vi "NM GlobalTest.vi"() -> ()   [LabVIEW 2010] (continued)
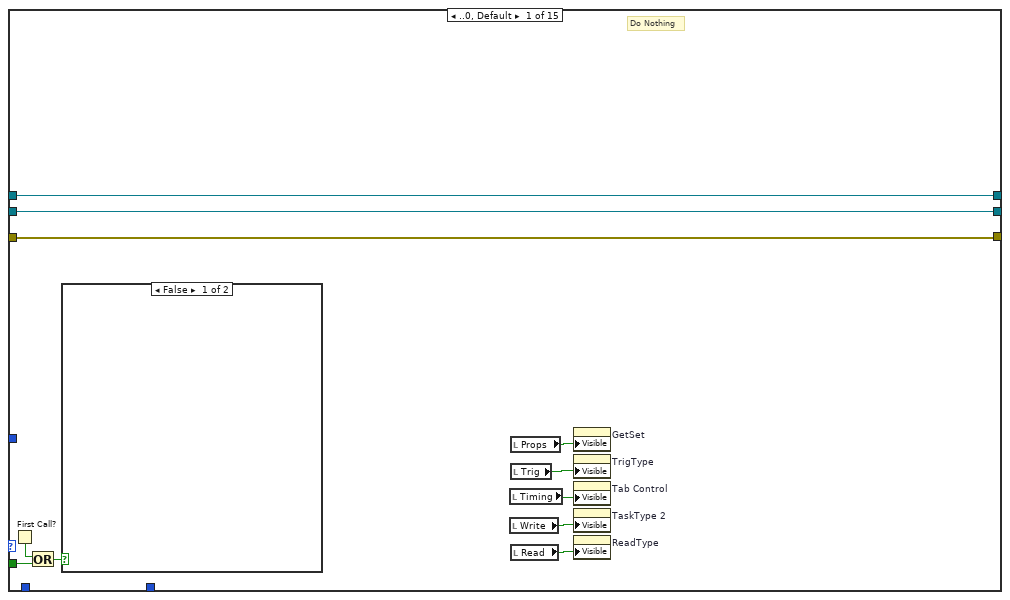
[diagram p2: hidden frame]
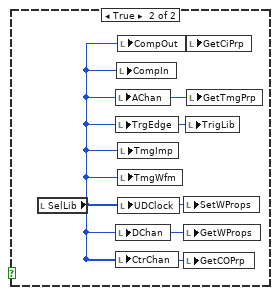
[diagram p3: hidden frame]
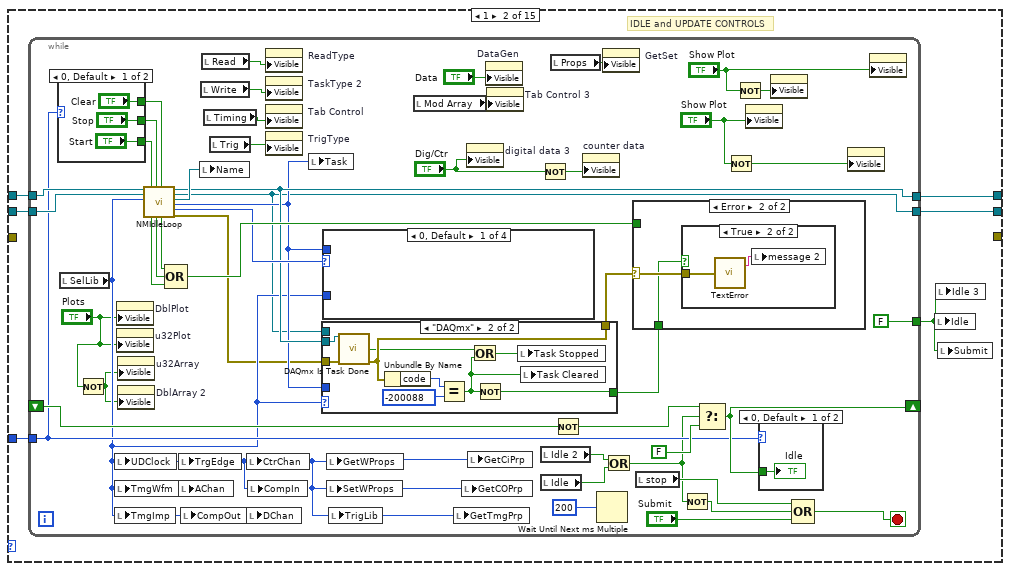
[diagram p4: hidden frame]
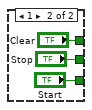
[diagram p5: hidden frame]
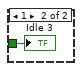
[diagram p6: hidden frame]
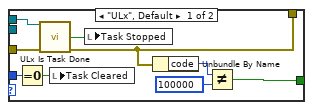
[diagram p7: hidden frame]
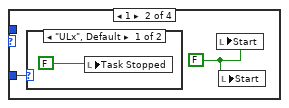
[diagram p8: hidden frame]
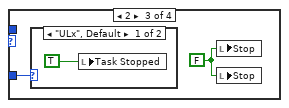
[diagram p10: hidden frame]
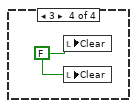
[diagram p12: hidden frame]
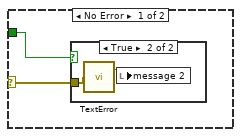
[diagram p13: hidden frame]
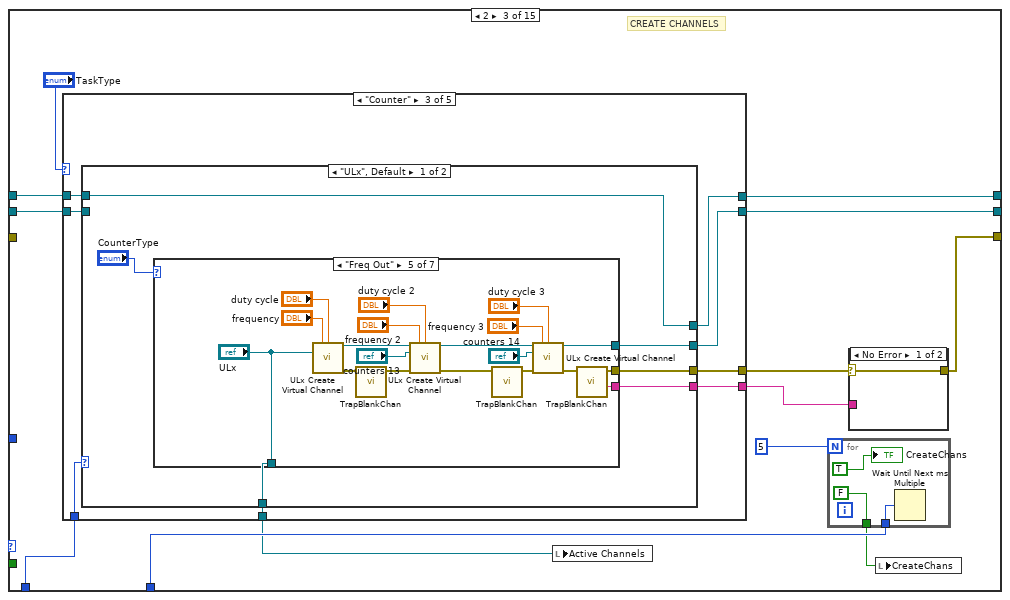
[diagram p16: hidden frame]
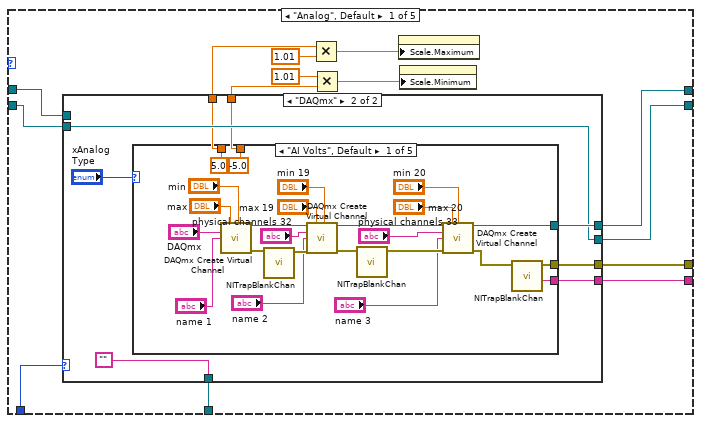
[diagram p17: hidden frame]
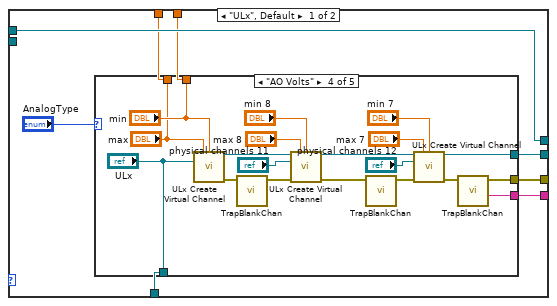
[diagram p18: hidden frame]
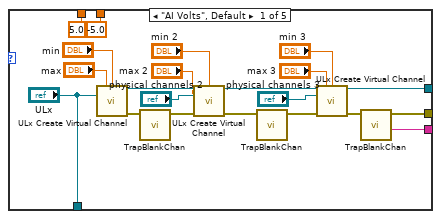
[diagram p19: hidden frame]
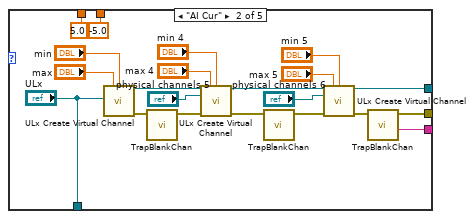
[diagram p20: hidden frame]
                                }
                                }
                                "Rate" <- w4838
                              }
                              frame 6 {
                                n979 = case shown="\"DAQmx\"" w4864 {
                                tunnel: w4863 -> [w4865 w4872]
                                tunnel: [w4865 w4871] -> w4862
                                tunnel: w4861 -> [w4866 w4870]
                                tunnel: [w4866 w4870] -> w4860
                                tunnel: w4859 -> [w4867 w4869]
                                tunnel: [w4867 w4868] -> w4858
                                frame "ULx", Default {
                                }
                                frame "DAQmx" {
                                n980 = property class="DAQmx Timing"(reference=w4869, error in=w4872) -> (reference out=w4868:refnum<k21>, error out=w4871:errorcluster, "SampClk.UnderflowBehavior"=→"SampClk.UnderflowBehavior":i32)
                                }
                                }
                              }
                            }
                          }
                        }
                        frame "AI" {
                          n981 = case shown="True" "Units" {
                            tunnel: w4905 -> [w4908 w4915]
                            tunnel: w4904 -> [w4907 w4914]
                            tunnel: w4903 -> [w4906 w4913]
                            tunnel: w4902 -> [_ w4912]
                            tunnel: [w4908 w4911] -> w4901
                            tunnel: [w4907 w4910] -> w4900
                            tunnel: [w4906 w4909] -> w4899
                            frame False {
                            }
                            frame True {
                              n982 = stacked-sequence {
                                seq-local: [w4919 _] -> [_ w4931]
                                seq-local: [w4918 _] -> [_ w4930]
                                seq-local: [w4917 _] -> [_ w4929]
                                tunnel: w4915 -> [w4922 _]
                                tunnel: w4914 -> [w4921 _]
                                tunnel: w4913 -> [w4920 _]
                                tunnel: w4912 -> [w4916 w4935]
                                tunnel: [_ w4934] -> w4911
                                tunnel: [_ w4933] -> w4910
                                tunnel: [_ w4932] -> w4909
                                frame #0 {
                                n983 = case shown="\"ULx\", Default" w4916 {
                                tunnel: w4921 -> [w4923 w4928]
                                tunnel: [w4924 w4927] -> w4917
                                tunnel: [w4923 w4928] -> w4918
                                tunnel: [w4925 w4926] -> w4919
                                tunnel: w4922 -> [w4925 w4926]
                                tunnel: w4920 -> [w4924 w4927]
                                frame "ULx", Default {
                                }
                                frame "DAQmx" {
                                }
                                }
                                }
                                frame #1 {
                                n984 = case shown="\"ULx\", Default" w4935 {
                                tunnel: w4930 -> [w4940 w4947]
                                tunnel: [w4936 w4945] -> w4932
                                tunnel: [w4937 w4947] -> w4933
                                tunnel: [w4941 w4943] -> w4934
                                tunnel: w4931 -> [w4941 w4944]
                                tunnel: w4929 -> [w4938 w4946]
                                frame "ULx", Default {
                                n985 = call "TempUnits.vi"("error in (no error)"=w4938, "task in"=w4940) -> ("error out"=w4936:errorcluster, "Temp.Units"=→"Channel.AI.Temp.Units":i32, "task out"=w4937:refnum<k24>)  [unwired: 1 in]
                                }
                                frame "DAQmx" {
                                n986 = property class="DAQmx Channel"(reference=w4944, error in=w4946) -> (reference out=w4943:refnum<k21>, error out=w4945:errorcluster, "AI.Temp.Units"=→"DAQmx AI.Temp.Units":i32)
                                }
                                }
                                }
                              }
                            }
                          }
                        }
                        frame "CI" {
                          n987 = stacked-sequence {
                            seq-local: [w4957 _] -> [_ w4974]
                            seq-local: [w4955 _] -> [_ w4973]
                            seq-local: [w4956 _] -> [_ w4972]
                            tunnel: w4954 -> [w4960 _]
                            tunnel: w4953 -> [w4955 _]
                            tunnel: w4952 -> [w4959 _]
                            tunnel: [_ w4977] -> w4951
                            tunnel: [_ w4976] -> w4950
                            tunnel: [_ w4975] -> w4949
                            tunnel: w4948 -> [w4958 w4971]
                            frame #0 {
                              n988 = case shown="\"ULx\", Default" w4958 {
                                tunnel: w4960 -> [w4961 w4969]
                                tunnel: w4959 -> [w4962 w4968]
                                tunnel: [w4962 w4967] -> w4957
                                tunnel: [w4961 w4966] -> w4956
                                frame "ULx", Default {
                                }
                                frame "DAQmx" {
                                n989 = property class="DAQmx Channel"(reference=w4968, error in=w4969) -> (reference out=w4967:refnum<k21>, error out=w4966:errorcluster, "CI.Max"=→"Max":dbl, "CI.Min"=→"Min":dbl, "CI.MeasType"=→"MeasType":i32)
                                }
                              }
                            }
                            frame #1 {
                              n990 = case shown="\"ULx\", Default" w4971 {
                                tunnel: ["CIType" "GetmxCIPrp"] -> w4970
                                frame "ULx", Default {
                                }
                                frame "DAQmx" {
                                }
                              }
                              n991 = case shown="\"Edges\"" w4970 {
                                tunnel: w4972 -> [w4986 w5010 w5038 w5077]
                                tunnel: w4973 -> [w4984 w5011 w5035 w5076]
                                tunnel: [w4981 w5009 w5036 w5075] -> w4977
                                tunnel: [w4985 w5007 w5037 w5073] -> w4976
                                tunnel: [w4983 w5008 w5034 w5074] -> w4975
                                tunnel: w4971 -> [w4982 w5012 w5033 w5072]
                                tunnel: w4974 -> [w4980 w5006 w5032 w5071]
                                frame "Frequency", Default {
                                n992 = case shown="\"ULx\", Default" w4982 {
                                tunnel: w4986 -> [w4992 w5005]
                                tunnel: [w4990 w4996] -> w4985
                                tunnel: w4984 -> [w4993 w5003]
                                tunnel: [w4991 w5003] -> w4983
                                tunnel: w4980 -> [w4994 w5004]
                                tunnel: [w4994 w4995] -> w4981
                                frame "ULx", Default {
                                n993 = call "CIFreqProps.vi"("task in"=w4993, "error in (no error)"=w4992) -> ("task out"=w4991:refnum<k24>, "StartingEdge"=→"StartingEdge":i32, "Units"=→"Units":i32, "error out"=w4990:errorcluster, "MeasurementTime"=→"MeasurementTime":dbl)  [unwired: 1 in]
                                }
                                frame "DAQmx" {
                                n994 = property class="DAQmx Channel"(reference=w5004, error in=w5005) -> (reference out=w4995:refnum<k21>, error out=w4996:errorcluster, "CI.Freq.Units"=→"Units":i32, "CI.Freq.Term"=→"Term":tag, "CI.Freq.StartingEdge"=→"StartingEdge":i32, "CI.Freq.MeasMeth"=→"Method":i32, "CI.Freq.MeasTime"=→"MeasTime":dbl, "CI.Freq.Div"=→"Divisor":u32)
                                }
                                }
                                }
                                frame "Period" {
                                n995 = case shown="\"ULx\", Default" w5012 {
                                tunnel: w5010 -> [w5017 w5031]
                                tunnel: [w5016 w5030] -> w5007
                                tunnel: w5011 -> [w5019 w5027]
                                tunnel: [w5018 w5027] -> w5008
                                tunnel: w5006 -> [w5020 w5029]
                                tunnel: [w5020 w5028] -> w5009
                                frame "ULx", Default {
                                n996 = call "CIPeriodProps.vi"("task in"=w5019, "error in (no error)"=w5017) -> ("task out"=w5018:refnum<k24>, "StartingEdge"=→"StartingEdge":i32, "Units"=→"Units":i32, "error out"=w5016:errorcluster, "MeasurementTime"=→"MeasurementTime":dbl)  [unwired: 1 in]
                                }
                                frame "DAQmx" {
                                n997 = property class="DAQmx Channel"(reference=w5029, error in=w5031) -> (reference out=w5028:refnum<k21>, error out=w5030:errorcluster, "CI.Period.Units"=→"Units":i32, "CI.Period.Term"=→"Term":tag, "CI.Period.StartingEdge"=→"StartingEdge":i32, "CI.Period.MeasMeth"=→"Method":i32, "CI.Period.MeasTime"=→"MeasTime":dbl, "CI.Period.Div"=→"Divisor":u32)
                                }
                                }
                                }
                                frame "Edges" {
                                n998 = case shown="\"ULx\", Default" w5033 {
                                tunnel: w5038 -> [w5059 w5070]
                                tunnel: [w5041 w5068] -> w5037
                                tunnel: w5035 -> [w5060 w5066]
                                tunnel: [w5042 w5066] -> w5034
                                tunnel: w5032 -> [w5061 w5069]
                                tunnel: [w5061 w5067] -> w5036
                                frame "ULx", Default {
                                n999 = call "CIEdgesProps.vi"("task in"=w5060, "error in (no error)"=w5059) -> ("task out"=w5048:refnum<k24>, "Edge"=→"Edge":i32, "InitialCount"=→"InitialCount":u32, "error out"=w5047:errorcluster, "Direction"=→"MccDirection":i32, "Gate Function"=→"Gate Function":i32)
                                n1000 = call "CtrCntrl.vi"("error in (no error)"=w5047, ".NET Refnum"=w5048) -> ("InvertGate"=→"InvertGate":bool, "Recycle"=→"Recycle":bool, "error out"=w5043:errorcluster, ".NET Refnum 2"=w5044:refnum<k24>, "OutputVal1"=→"Val 1":u64, "MinLimit"=→"Min":u64, "OutputVal0"=→"Val 0":u64, "MaxLimit"=→"Max":u64, "OutputOn"=→"Output":bool, "RangeLimitOn"=→"Range Limit":bool)
                                n1001 = call "CtrProps.vi"("error in (no error)"=w5043, ".NET Refnum 2"=w5044) -> ("InitialState"=→"InitialState":i32, "ClearOnRead"=→"ClearOnRead":bool, "error out"=w5041:errorcluster, ".NET Refnum"=w5042:refnum<k24>)  [unwired: 6 in]
                                }
                                frame "DAQmx" {
                                n1002 = property class="DAQmx Channel"(reference=w5069, error in=w5070) -> (reference out=w5067:refnum<k21>, error out=w5068:errorcluster, "CI.CountEdges.Term"=→"Term":tag, "CI.CountEdges.Dir"=→"Direction":i32, "CI.CountEdges.InitialCnt"=→"InitialCnt":u32, "CI.CountEdges.ActiveEdge"=→"ActiveEdge":i32)
                                }
                                }
                                }
                                frame "Encoder" {
                                n1003 = case shown="\"ULx\", Default" w5072 {
                                tunnel: w5077 -> [w5086 w5100]
                                tunnel: [w5078 w5099] -> w5073
                                tunnel: w5076 -> [w5085 w5098]
                                tunnel: [w5079 w5098] -> w5074
                                tunnel: w5071 -> [w5087 w5102]
                                tunnel: [w5087 w5101] -> w5075
                                frame "ULx", Default {
                                n1004 = call "CIEncoderProps.vi"("task in"=w5085, "error in (no error)"=w5086) -> ("Units"=→"Units":i32, "DecodingType"=→"DecodingType":i32, "task out"=w5079:refnum<k24>, "PulsesPerRevolution"=→"PulsesPerRev":i32, "InitialAngle"=→"InitialAngle":dbl, "ZIndexMode"=→"ZIndexMode":i32, "error out"=w5078:errorcluster)  [unwired: 2 in]
                                }
                                frame "DAQmx" {
                                n1005 = property class="DAQmx Channel"(reference=w5102, error in=w5100) -> (reference out=w5101:refnum<k21>, error out=w5099:errorcluster, "CI.AngEncoder.Units"=→"Units":i32, "CI.AngEncoder.PulsesPerRev"=→"PulsesPerRev":u32, "CI.AngEncoder.InitialAngle"=→"InitialAngle":dbl, "CI.Encoder.DecodingType"=→"Type":i32, "CI.Encoder.AInputTerm"=→"AInputTerm":tag, "CI.Encoder.BInputTerm"=→"BInputTerm":tag, "CI.Encoder.ZInputTerm"=→"ZInputTerm":tag, "CI.Encoder.ZIndexEnable"=→"ZIndex":bool, "CI.Encoder.ZIndexVal"=→"Value":dbl, "CI.Encoder.ZIndexPhase"=→"Phase":i32)
                                }
                                }
                                }
                              }
                            }
                          }
                        }
                        frame "CO" {
                          n1006 = case shown="\"ULx\", Default" w5103 {
                            tunnel: w5108 -> [w5119 w5130]
                            tunnel: [w5116 w5121] -> w5104
                            tunnel: [w5117 w5130] -> w5105
                            tunnel: [w5120 w5122] -> w5106
                            tunnel: w5109 -> [w5120 w5127]
                            tunnel: w5107 -> [w5118 w5126]
                            frame "ULx", Default {
                              n1007 = call "COPulseProps.vi"("task in"=w5119, "error in (no error)"=w5118) -> ("DutyCycle"=→"DutyCycle":dbl, "HighTicks"=→"HighTicks":u32, "HighTime"=→"HighTime":dbl, "task out"=w5117:refnum<k24>, "LowTicks"=→"LowTicks":u32, "Frequency"=→"Frequency":dbl, "LowTime"=→"LowTime":dbl, "error out"=w5116:errorcluster)  [unwired: 1 in]
                            }
                            frame "DAQmx" {
                              n1008 = property class="DAQmx Channel"(reference=w5127, error in=w5126) -> (reference out=w5124:refnum<k21>, error out=w5123:errorcluster, "CO.OutputType"=→"OutputType":i32, "CO.Pulse.IdleState"=→"IdleState":i32)
                              n1009 = case shown="\"Freq\", Default" "mxCOType" {
                                tunnel: w5124 -> [w5138 w5143 w5152]
                                tunnel: w5123 -> [w5137 w5146 w5153]
                                tunnel: [w5136 w5144 w5151] -> w5122
                                tunnel: [w5135 w5145 w5150] -> w5121
                                frame "Freq", Default {
                                n1010 = property class="DAQmx Channel"(reference=w5138, error in=w5137) -> (reference out=w5136:refnum<k21>, error out=w5135:errorcluster, "CO.Pulse.DutyCyc"=→"DutyCyc":dbl, "CO.Pulse.Freq.Units"=→"Freq.Units":i32, "CO.Pulse.Freq"=→"Freq":dbl, "CO.Pulse.Freq.InitialDelay"=→"Freq.Delay":dbl)
                                }
                                frame "Time" {
                                n1011 = property class="DAQmx Channel"(reference=w5143, error in=w5146) -> (reference out=w5144:refnum<k21>, error out=w5145:errorcluster, "CO.Pulse.Time.Units"=→"Time.Units":i32, "CO.Pulse.HighTime"=→"HighTime":dbl, "CO.Pulse.LowTime"=→"LowTime":dbl, "CO.Pulse.Time.InitialDelay"=→"Time.Delay":dbl)
                                }
                                frame "Ticks" {
                                n1012 = property class="DAQmx Channel"(reference=w5152, error in=w5153) -> (reference out=w5151:refnum<k21>, error out=w5150:errorcluster, "CO.Pulse.HighTicks"=→"HighTicks":u32, "CO.Pulse.LowTicks"=→"LowTicks":u32, "CO.Pulse.Ticks.InitialDelay"=→"Ticks.Delay":u32)
                                }
                              }
                            }
                          }
                        }
                      }
                    }
                  }
                }
                frame "Set Properties" {
                  n1013 = case shown="\"Write\"" "SetLev" {
                    tunnel: w5161 -> [w5169 w5257 _ w5379 _ w5475 w5725]
                    tunnel: w5160 -> [w5167 w5263 w5371 w5376 w5472 w5480 w5722]
                    tunnel: [w5166 w5260 w5371 w5375 w5472 w5479 w5720] -> w5159
                    tunnel: [w5165 w5259 w5370 w5374 w5471 w5477 w5719] -> w5158
                    tunnel: w5157 -> [w5164 w5262 w5370 w5377 w5471 w5474 w5723]
                    tunnel: w5156 -> [w5163 w5261 w5369 w5378 w5470 w5473 w5724]
                    tunnel: [w5162 w5258 w5369 w5373 w5470 w5478 w5718] -> w5154
                    frame "Read", Default {
                      n1014 = for {
                        N: 3 -> [_]
                        tunnel: w5169 -> [w5175]
                        shift-right: [w5178] -> w5166
                        shift-left: w5167 -> [w5172]
                        shift-right: [w5177] -> w5165
                        shift-left: w5164 -> [w5171]
                        shift-right: [w5176] -> w5162
                        shift-left: w5163 -> [w5170]
                        i -> [w5174]
                        n1015 = case shown="0, Default" w5174 {
                          tunnel: [w5179 w5183 w5187] -> w5173
                          frame 0, Default {
                            n1016 = Select(t=1, s="Auto", f=0) -> (s? t:f=w5179:i32)
                          }
                          frame 1 {
                            n1017 = Select(t=2, s="OWrite", f=0) -> (s? t:f=w5183:i32)
                          }
                          frame 2 {
                            n1018 = Select(t=3, s="ReadAll 2", f=0) -> (s? t:f=w5187:i32)
                          }
                        }
                        n1019 = case shown="3" w5173 {
                          tunnel: w5172 -> [w5193 w5202 w5217 w5244]
                          tunnel: w5171 -> [w5192 w5201 w5221 w5243]
                          tunnel: w5170 -> [w5191 w5200 w5223 w5242]
                          tunnel: [w5193 w5199 w5216 w5240] -> w5178
                          tunnel: [w5192 w5198 w5220 w5241] -> w5177
                          tunnel: [w5191 w5197 w5222 w5239] -> w5176
                          tunnel: w5175 -> [_ w5196 w5218 w5237]
                          frame 0, Default {
                          }
                          frame 1 {
                            n1020 = case shown="\"ULx\", Default" w5196 {
                              tunnel: w5201 -> [w5203 w5214]
                              tunnel: [w5205 w5212] -> w5197
                              tunnel: [w5204 w5214] -> w5198
                              tunnel: [w5208 w5211] -> w5199
                              tunnel: w5202 -> [w5208 w5210]
                              tunnel: w5200 -> [w5206 w5213]
                              tunnel: "Read.AutoStart" -> [w5207 w5209]
                              frame "ULx", Default {
                                n1021 = call "SetReadAutostart.vi"("error in (no error)"=w5206, "Read.AutoStart"=w5207, "task in"=w5203) -> ("error out"=w5205:errorcluster, "task out"=w5204:refnum<k24>)
                              }
                              frame "DAQmx" {
                                n1022 = property class="DAQmx Read"(reference=w5210, error in=w5213, "AutoStart"=w5209) -> (reference out=w5211:refnum<k21>, error out=w5212:errorcluster)
                              }
                            }
                            n1023 = local write "Auto"(FALSE ("Auto")) -> ()
                          }
                          frame 2 {
                            n1024 = case shown="\"ULx\", Default" w5218 {
                              tunnel: w5223 -> [w5224 w5233]
                              tunnel: [w5224 w5232] -> w5222
                              tunnel: w5221 -> [w5225 w5229]
                              tunnel: [w5225 w5229] -> w5220
                              tunnel: w5217 -> [w5226 w5231]
                              tunnel: [w5226 w5230] -> w5216
                              tunnel: "Overwrite" -> [_ w5228]
                              frame "ULx", Default {
                              }
                              frame "DAQmx" {
                                n1025 = case shown="False" w5228 {
                                tunnel: [w5234 w5235] -> w5227
                                frame False {
                                w5234 = 10159 items=["Overwrite Unread Samples"=10252, "Do Not Overwrite Unread Samples"=10159] ("OverWrite")
                                }
                                frame True {
                                w5235 = 10252 items=["Overwrite Unread Samples"=10252, "Do Not Overwrite Unread Samples"=10159] ("OverWrite")
                                }
                                }
                                n1026 = property class="DAQmx Read"(reference=w5231, error in=w5233, "OverWrite"=w5227) -> (reference out=w5230:refnum<k21>, error out=w5232:errorcluster)
                              }
                            }
                            n1027 = local write "OWrite"(FALSE ("Auto 2")) -> ()
                          }
                          frame 3 {
                            n1028 = case shown="\"ULx\", Default" w5237 {
                              tunnel: w5242 -> [w5249 w5256]
                              tunnel: [w5248 w5255] -> w5239
                              tunnel: w5243 -> [w5247 w5252]
                              tunnel: [w5246 w5252] -> w5241
                              tunnel: w5244 -> [w5250 w5254]
                              tunnel: [w5250 w5253] -> w5240
                              tunnel: "ReadAllAvailSamp" -> [w5245 w5251]
                              frame "ULx", Default {
                                n1029 = call "SetReadAllData.vi"("error in (no error)"=w5249, "Read.AllData"=w5245, "task in"=w5247) -> ("error out"=w5248:errorcluster, "task out"=w5246:refnum<k24>)
                              }
                              frame "DAQmx" {
                                n1030 = property class="DAQmx Read"(reference=w5254, error in=w5256, "ReadAllAvailSamp"=w5251) -> (reference out=w5253:refnum<k21>, error out=w5255:errorcluster)
                              }
                            }
                            n1031 = local write "ReadAll 2"(FALSE ("ReadAll 2")) -> ()
                          }
                        }
                      }
                    }
                    frame "Write" {
                      n1032 = for {
                        N: 4 -> [_]
                        shift-right: [w5269] -> w5260
                        shift-left: w5263 -> [w5271]
                        shift-right: [w5268] -> w5259
                        shift-left: w5262 -> [w5270]
                        shift-right: [w5272] -> w5258
                        shift-left: w5261 -> [w5273]
                        tunnel: w5257 -> [w5265]
                        i -> [w5267]
                        n1033 = case shown="0, Default" w5267 {
                          tunnel: [w5274 w5278 w5282 w5286] -> w5266
                          frame 0, Default {
                            n1034 = Select(t=1, s="WrtPos", f=0) -> (s? t:f=w5274:i32)
                          }
                          frame 1 {
                            n1035 = Select(t=2, s="Reg", f=0) -> (s? t:f=w5278:i32)
                          }
                          frame 2 {
                            n1036 = Select(t=3, s="Rel", f=0) -> (s? t:f=w5282:i32)
                          }
                          frame 3 {
                            n1037 = Select(t=4, s="Offset 3", f=0) -> (s? t:f=w5286:i32)
                          }
                        }
                        n1038 = case shown="4" w5266 {
                          tunnel: w5273 -> [w5290 w5301 w5319 w5339 w5356]
                          tunnel: [w5290 w5300 w5314 w5335 w5352] -> w5272
                          tunnel: w5271 -> [w5292 w5299 w5318 w5341 w5358]
                          tunnel: w5270 -> [w5291 w5298 w5317 w5340 w5357]
                          tunnel: [w5292 w5297 w5316 w5337 w5354] -> w5269
                          tunnel: [w5291 w5296 w5315 w5336 w5353] -> w5268
                          tunnel: w5265 -> [_ w5295 w5313 w5338 w5355]
                          frame 0, Default {
                          }
                          frame 1 {
                            n1039 = case shown="\"DAQmx\"" w5295 {
                              tunnel: w5298 -> [w5304 w5310]
                              tunnel: [w5305 w5309] -> w5300
                              tunnel: [w5303 w5310] -> w5296
                              tunnel: [w5307 w5308] -> w5297
                              tunnel: w5299 -> [w5307 w5308]
                              tunnel: w5301 -> [w5306 w5309]
                              tunnel: "CurrentWrite\nPosition (ULx)" -> [w5302 _]
                              frame "ULx", Default {
                                n1040 = call "SetCurWrtPos.vi"("error in (no error)"=w5306, "CurrentWritePosition"=w5302, "task in"=w5304) -> ("error out"=w5305:errorcluster, "task out"=w5303:refnum<k24>)
                              }
                              frame "DAQmx" {
                              }
                            }
                            n1041 = local write "WrtPos"(FALSE ("WrtPos")) -> ()
                          }
                          frame 2 {
                            n1042 = case shown="\"ULx\", Default" w5313 {
                              tunnel: w5319 -> [w5322 w5331]
                              tunnel: [w5321 w5327] -> w5314
                              tunnel: w5317 -> [w5323 w5330]
                              tunnel: [w5320 w5330] -> w5315
                              tunnel: w5318 -> [w5325 w5329]
                              tunnel: [w5325 w5328] -> w5316
                              tunnel: "Regenerate" -> [w5324 w5326]
                              frame "ULx", Default {
                                n1043 = call "SetWrtRegen.vi"("error in (no error)"=w5322, "Regenerate"=w5324, "task in"=w5323) -> ("error out"=w5321:errorcluster, "task out"=w5320:refnum<k24>)
                              }
                              frame "DAQmx" {
                                n1044 = case shown="True" w5326 {
                                tunnel: [w5333 w5334] -> w5332
                                frame False {
                                w5333 = 10158 items=["Allow Regeneration"=10097, "Do Not Allow Regeneration"=10158] ("RegenMode")
                                }
                                frame True {
                                w5334 = 10097 items=["Allow Regeneration"=10097, "Do Not Allow Regeneration"=10158] ("RegenMode")
                                }
                                }
                                n1045 = property class="DAQmx Write"(reference=w5329, error in=w5331, "RegenMode"=w5332) -> (reference out=w5328:refnum<k21>, error out=w5327:errorcluster)
                              }
                            }
                            n1046 = local write "Reg"(FALSE ("Reg")) -> ()
                          }
                          frame 3 {
                            n1047 = case shown="\"DAQmx\"" w5338 {
                              tunnel: w5339 -> [w5343 w5351]
                              tunnel: [w5343 w5347] -> w5335
                              tunnel: w5340 -> [w5342 w5350]
                              tunnel: [w5342 w5350] -> w5336
                              tunnel: w5341 -> [w5344 w5349]
                              tunnel: [w5344 w5348] -> w5337
                              frame "ULx", Default {
                              }
                              frame "DAQmx" {
                                n1048 = property class="DAQmx Write"(reference=w5349, error in=w5351, "RelativeTo"="RelativeTo") -> (reference out=w5348:refnum<k21>, error out=w5347:errorcluster)
                                n1049 = local write "Rel"(FALSE ("Rel")) -> ()
                              }
                            }
                          }
                          frame 4 {
                            n1050 = case shown="\"DAQmx\"" w5355 {
                              tunnel: w5356 -> [w5360 w5368]
                              tunnel: [w5360 w5364] -> w5352
                              tunnel: w5357 -> [w5359 w5367]
                              tunnel: [w5359 w5367] -> w5353
                              tunnel: w5358 -> [w5361 w5366]
                              tunnel: [w5361 w5365] -> w5354
                              frame "ULx", Default {
                              }
                              frame "DAQmx" {
                                n1051 = property class="DAQmx Write"(reference=w5366, error in=w5368, "Offset"="Offset") -> (reference out=w5365:refnum<k21>, error out=w5364:errorcluster)
                                n1052 = local write "Offset 3"(FALSE ("Rel")) -> ()
                              }
                            }
                          }
                        }
                      }
                    }
                    frame "Trigger" {
                    }
                    frame "Timing" {
                      n1053 = for {
                        N: 4 -> [_]
                        tunnel: w5379 -> [w5388]
                        shift-right: [w5384] -> w5375
                        shift-left: w5376 -> [w5385]
                        shift-right: [w5383] -> w5374
                        shift-left: w5377 -> [w5386]
                        shift-right: [w5382] -> w5373
                        shift-left: w5378 -> [w5387]
                        i -> [w5381]
                        n1054 = case shown="0, Default" w5381 {
                          tunnel: [w5389 w5393 w5397 w5401] -> w5380
                          frame 0, Default {
                            n1055 = Select(t=1, s="BurstIO 3", f=0) -> (s? t:f=w5389:i32)
                          }
                          frame 1 {
                            n1056 = Select(t=2, s="SingleIO 3", f=0) -> (s? t:f=w5393:i32)
                          }
                          frame 2 {
                            n1057 = Select(t=3, s="DIWord", f=0) -> (s? t:f=w5397:i32)
                          }
                          frame 3 {
                            n1058 = Select(t=4, s="DOWord 2", f=0) -> (s? t:f=w5401:i32)
                          }
                        }
                        n1059 = case shown="1" w5380 {
                          tunnel: w5388 -> [_ w5415 w5426 w5443 w5457]
                          tunnel: w5387 -> [w5405 w5414 w5427 w5442 w5458]
                          tunnel: w5386 -> [w5406 w5413 w5428 w5441 w5459]
                          tunnel: w5385 -> [w5407 w5412 w5429 w5440 w5460]
                          tunnel: [w5407 w5411 w5425 w5439 w5454] -> w5384
                          tunnel: [w5406 w5410 w5424 w5438 w5455] -> w5383
                          tunnel: [w5405 w5409 w5423 w5437 w5456] -> w5382
                          frame 0, Default {
                          }
                          frame 1 {
                            n1060 = case shown="\"ULx\", Default" w5415 {
                              tunnel: w5414 -> [w5416 w5420]
                              tunnel: [w5416 w5420] -> w5409
                              tunnel: w5413 -> [w5417 w5421]
                              tunnel: [w5417 w5421] -> w5410
                              tunnel: w5412 -> [w5418 w5419]
                              tunnel: [w5418 w5419] -> w5411
                              frame "ULx", Default {
                              }
                              frame "DAQmx" {
                              }
                            }
                            n1061 = local write "BurstIO 3"(FALSE ("BurstIO 3")) -> ()
                          }
                          frame 2 {
                            n1062 = case shown="\"ULx\", Default" w5426 {
                              tunnel: w5427 -> [w5431 w5434]
                              tunnel: [w5431 w5434] -> w5423
                              tunnel: w5428 -> [w5430 w5435]
                              tunnel: [w5430 w5435] -> w5424
                              tunnel: w5429 -> [w5432 w5433]
                              tunnel: [w5432 w5433] -> w5425
                              frame "ULx", Default {
                              }
                              frame "DAQmx" {
                              }
                            }
                            n1063 = local write "SingleIO 3"(FALSE ("SingleIO 2")) -> ()
                          }
                          frame 3 {
                            n1064 = case shown="\"ULx\", Default" w5443 {
                              tunnel: w5442 -> [w5448 w5451]
                              tunnel: [w5447 w5451] -> w5437
                              tunnel: w5441 -> [w5446 w5452]
                              tunnel: [w5445 w5452] -> w5438
                              tunnel: w5440 -> [w5449 w5450]
                              tunnel: [w5449 w5450] -> w5439
                              frame "ULx", Default {
                                n1065 = call "SetDIWord.vi"("error in (no error)"=w5448, "DIWord"="DIWord", "task in"=w5446) -> ("error out"=w5447:errorcluster, "task out"=w5445:refnum<k24>)
                              }
                              frame "DAQmx" {
                              }
                            }
                            n1066 = local write "DIWord"(FALSE ("DIWord")) -> ()
                          }
                          frame 4 {
                            n1067 = case shown="\"ULx\", Default" w5457 {
                              tunnel: w5458 -> [w5465 w5468]
                              tunnel: [w5464 w5468] -> w5456
                              tunnel: w5459 -> [w5463 w5469]
                              tunnel: [w5462 w5469] -> w5455
                              tunnel: w5460 -> [w5466 w5467]
                              tunnel: [w5466 w5467] -> w5454
                              frame "ULx", Default {
                                n1068 = call "SetDOWord.vi"("error in (no error)"=w5465, "DOWord"="DOWord", "task in"=w5463) -> ("error out"=w5464:errorcluster, "task out"=w5462:refnum<k24>)
                              }
                              frame "DAQmx" {
                              }
                            }
                            n1069 = local write "DOWord 2"(FALSE ("DOWord 2")) -> ()
                          }
                        }
                      }
                    }
                    frame "AI" {
                    }
                    frame "CI" {
                      n1070 = for {
                        N: 11 -> [_]
                        tunnel: w5475 -> [w5489]
                        shift-right: [w5485] -> w5478
                        shift-left: w5473 -> [w5486]
                        shift-right: [w5483] -> w5477
                        shift-left: w5474 -> [w5484]
                        shift-right: [w5487] -> w5479
                        shift-left: w5480 -> [w5488]
                        i -> [w5482]
                        n1071 = case shown="10" w5482 {
                          tunnel: [w5674 w5678 w5685 w5686 w5690 w5694 w5698 w5702 w5706 w5710 w5714] -> w5481
                          frame 0, Default {
                            n1072 = Select(t=1, s="MinMax", f=0) -> (s? t:f=w5674:i32)
                          }
                          frame 1 {
                            n1073 = Select(t=2, s="Set Dir", f=0) -> (s? t:f=w5678:i32)
                          }
                          frame 2 {
                            n1074 = Select(t=3, s="Gate", f=0) -> (s? t:f=w5685:i32)
                          }
                          frame 3 {
                            n1075 = Select(t=4, s="ClearOnRead 2", f=0) -> (s? t:f=w5686:i32)
                          }
                          frame 4 {
                            n1076 = Select(t=5, s="RangeLimit", f=0) -> (s? t:f=w5690:i32)
                          }
                          frame 5 {
                            n1077 = Select(t=6, s="OutputOn", f=0) -> (s? t:f=w5694:i32)
                          }
                          frame 6 {
                            n1078 = Select(t=7, s="NoRecycle", f=0) -> (s? t:f=w5698:i32)
                          }
                          frame 7 {
                            n1079 = Select(t=8, s="Invert Gate", f=0) -> (s? t:f=w5702:i32)
                          }
                          frame 8 {
                            n1080 = Select(t=9, s="Mcc Direction", f=0) -> (s? t:f=w5706:i32)
                          }
                          frame 9 {
                            n1081 = Select(t=10, s="Mcc Edge", f=0) -> (s? t:f=w5710:i32)
                          }
                          frame 10 {
                            n1082 = Select(t=11, s="Init State", f=0) -> (s? t:f=w5714:i32)
                          }
                        }
                        n1083 = case shown="11" w5481 {
                          tunnel: w5489 -> [_ w5496 w5510 w5529 w5544 w5560 w5576 w5596 w5616 w5629 w5645 w5661]
                          tunnel: w5488 -> [w5492 w5499 w5514 w5532 w5548 w5564 w5582 w5600 w5615 w5632 w5648 w5664]
                          tunnel: [w5492 w5495 w5513 w5528 w5547 w5563 w5581 w5599 w5612 w5628 w5644 w5660] -> w5487
                          tunnel: w5486 -> [w5490 w5497 w5516 w5530 w5545 w5561 w5579 w5597 w5611 w5630 w5646 w5662]
                          tunnel: [w5490 w5493 w5511 w5526 w5542 w5558 w5577 w5594 w5610 w5626 w5642 w5658] -> w5485
                          tunnel: w5484 -> [w5491 w5498 w5515 w5531 w5546 w5562 w5580 w5598 w5614 w5631 w5647 w5663]
                          tunnel: [w5491 w5494 w5512 w5527 w5543 w5559 w5578 w5595 w5613 w5627 w5643 w5659] -> w5483
                          frame 0, Default {
                          }
                          frame 1 {
                            n1084 = case shown="\"ULx\", Default" w5496 {
                              tunnel: w5499 -> [w5502 w5509]
                              tunnel: [w5502 w5508] -> w5495
                              tunnel: w5497 -> [w5500 w5507]
                              tunnel: [w5500 w5506] -> w5493
                              tunnel: w5498 -> [w5501 w5505]
                              tunnel: [w5501 w5505] -> w5494
                              frame "ULx", Default {
                              }
                              frame "DAQmx" {
                                n1085 = property class="DAQmx Channel"(reference=w5509, error in=w5507, "CI.Max"="Max", "CI.Min"="Min") -> (reference out=w5508:refnum<k21>, error out=w5506:errorcluster)
                              }
                            }
                          }
                          frame 2 {
                            n1086 = case shown="\"ULx\", Default" w5510 {
                              tunnel: w5514 -> [w5518 w5525]
                              tunnel: [w5518 w5524] -> w5513
                              tunnel: w5516 -> [w5519 w5523]
                              tunnel: [w5519 w5522] -> w5511
                              tunnel: w5515 -> [w5517 w5521]
                              tunnel: [w5517 w5521] -> w5512
                              frame "ULx", Default {
                              }
                              frame "DAQmx" {
                                n1087 = property class="DAQmx Channel"(reference=w5525, error in=w5523, "CI.CountEdges.Dir"="Direction") -> (reference out=w5524:refnum<k21>, error out=w5522:errorcluster)
                              }
                            }
                          }
                          frame 3 {
                            n1088 = case shown="\"ULx\", Default" w5529 {
                              tunnel: w5532 -> [w5538 w5540]
                              tunnel: [w5538 w5540] -> w5528
                              tunnel: w5530 -> [w5537 w5539]
                              tunnel: [w5534 w5539] -> w5526
                              tunnel: w5531 -> [w5536 w5541]
                              tunnel: [w5535 w5541] -> w5527
                              frame "ULx", Default {
                                n1089 = property class="IOTask"(reference=w5536, error in=w5537, "Channel.CI.CountEdges.GateFunction"="Gate Function 2") -> (reference out=w5535:refnum<k24>, error out=w5534:errorcluster)
                              }
                              frame "DAQmx" {
                              }
                            }
                          }
                          frame 4 {
                            n1090 = case shown="\"ULx\", Default" w5544 {
                              tunnel: w5548 -> [w5554 w5556]
                              tunnel: [w5554 w5556] -> w5547
                              tunnel: w5545 -> [w5552 w5555]
                              tunnel: [w5551 w5555] -> w5542
                              tunnel: w5546 -> [w5550 w5557]
                              tunnel: [w5549 w5557] -> w5543
                              frame "ULx", Default {
                                n1091 = property class="IOTask"(reference=w5550, error in=w5552, "Channel.CI.CountEdges.ClearOnRead"="ClearOnRead") -> (reference out=w5549:refnum<k24>, error out=w5551:errorcluster)
                              }
                              frame "DAQmx" {
                              }
                            }
                          }
                          frame 5 {
                            n1092 = case shown="\"ULx\", Default" w5560 {
                              tunnel: w5564 -> [w5572 w5574]
                              tunnel: [w5572 w5574] -> w5563
                              tunnel: w5561 -> [w5570 w5573]
                              tunnel: [w5569 w5573] -> w5558
                              tunnel: w5562 -> [w5568 w5575]
                              tunnel: [w5567 w5575] -> w5559
                              frame "ULx", Default {
                                n1093 = property class="IOTask"(reference=w5568, error in=w5570, "Channel.CI.CountEdges.RangeLimitOn"="RangeLimOn", "Channel.CI.CountEdges.Registers.MaxLimit"="MaxLimit", "Channel.CI.CountEdges.Registers.MinLimit"="MinLimit") -> (reference out=w5567:refnum<k24>, error out=w5569:errorcluster)
                              }
                              frame "DAQmx" {
                              }
                            }
                          }
                          frame 6 {
                            n1094 = case shown="\"ULx\", Default" w5576 {
                              tunnel: w5582 -> [w5590 w5592]
                              tunnel: [w5590 w5592] -> w5581
                              tunnel: w5579 -> [w5588 w5591]
                              tunnel: [w5587 w5591] -> w5577
                              tunnel: w5580 -> [w5586 w5593]
                              tunnel: [w5585 w5593] -> w5578
                              frame "ULx", Default {
                                n1095 = property class="IOTask"(reference=w5586, error in=w5588, "Channel.CI.CountEdges.OutputOn"="Output", "Channel.CI.CountEdges.Registers.OutputVal0"="Out0", "Channel.CI.CountEdges.Registers.OutputVal1"="Out1") -> (reference out=w5585:refnum<k24>, error out=w5587:errorcluster)
                              }
                              frame "DAQmx" {
                              }
                            }
                          }
                          frame 7 {
                            n1096 = case shown="\"ULx\", Default" w5596 {
                              tunnel: w5600 -> [w5606 w5608]
                              tunnel: [w5606 w5608] -> w5599
                              tunnel: w5597 -> [w5604 w5607]
                              tunnel: [w5603 w5607] -> w5594
                              tunnel: w5598 -> [w5602 w5609]
                              tunnel: [w5601 w5609] -> w5595
                              frame "ULx", Default {
                                n1097 = property class="IOTask"(reference=w5602, error in=w5604, "Channel.CI.CountEdges.Recycle"="Recycle") -> (reference out=w5601:refnum<k24>, error out=w5603:errorcluster)
                              }
                              frame "DAQmx" {
                              }
                            }
                          }
                          frame 8 {
                            n1098 = case shown="\"ULx\", Default" w5616 {
                              tunnel: w5611 -> [w5622 w5624]
                              tunnel: [w5620 w5623] -> w5613
                              tunnel: [w5619 w5624] -> w5610
                              tunnel: w5615 -> [w5617 w5625]
                              tunnel: [w5617 w5625] -> w5612
                              tunnel: w5614 -> [w5618 w5623]
                              frame "ULx", Default {
                                n1099 = property class="IOTask"(reference=w5618, error in=w5622, "Channel.CI.CountEdges.InvertGate"="Invert Gate") -> (reference out=w5620:refnum<k24>, error out=w5619:errorcluster)
                              }
                              frame "DAQmx" {
                              }
                            }
                          }
                          frame 9 {
                            n1100 = case shown="\"ULx\", Default" w5629 {
                              tunnel: w5630 -> [w5638 w5640]
                              tunnel: [w5637 w5639] -> w5627
                              tunnel: [w5636 w5640] -> w5626
                              tunnel: w5632 -> [w5634 w5641]
                              tunnel: [w5634 w5641] -> w5628
                              tunnel: w5631 -> [w5635 w5639]
                              frame "ULx", Default {
                                n1101 = property class="IOTask"(reference=w5635, error in=w5638, "Channel.CI.CountEdges.CountDirection"="MccDirection") -> (reference out=w5637:refnum<k24>, error out=w5636:errorcluster)
                              }
                              frame "DAQmx" {
                              }
                            }
                          }
                          frame 10 {
                            n1102 = case shown="\"ULx\", Default" w5645 {
                              tunnel: w5646 -> [w5654 w5656]
                              tunnel: [w5653 w5655] -> w5643
                              tunnel: [w5652 w5656] -> w5642
                              tunnel: w5648 -> [w5650 w5657]
                              tunnel: [w5650 w5657] -> w5644
                              tunnel: w5647 -> [w5651 w5655]
                              frame "ULx", Default {
                                n1103 = property class="IOTask"(reference=w5651, error in=w5654, "Channel.CI.CountEdges.Edge"="MccEdge") -> (reference out=w5653:refnum<k24>, error out=w5652:errorcluster)
                              }
                              frame "DAQmx" {
                              }
                            }
                          }
                          frame 11 {
                            n1104 = case shown="\"ULx\", Default" w5661 {
                              tunnel: w5662 -> [w5670 w5672]
                              tunnel: [w5669 w5671] -> w5659
                              tunnel: [w5668 w5672] -> w5658
                              tunnel: w5664 -> [w5666 w5673]
                              tunnel: [w5666 w5673] -> w5660
                              tunnel: w5663 -> [w5667 w5671]
                              frame "ULx", Default {
                                n1105 = property class="IOTask"(reference=w5667, error in=w5670, "Channel.CI.CountEdges.OutputInitialState"="Initial State") -> (reference out=w5669:refnum<k24>, error out=w5668:errorcluster)
                              }
                              frame "DAQmx" {
                              }
                            }
                          }
                        }
                      }
                    }
                    frame "CO" {
                      n1106 = for {
                        N: 2 -> [_]
                        tunnel: w5725 -> [w5731]
                        shift-right: [w5734] -> w5720
                        shift-left: w5722 -> [w5728]
                        shift-right: [w5733] -> w5719
                        shift-left: w5723 -> [w5727]
                        shift-right: [w5732] -> w5718
                        shift-left: w5724 -> [w5726]
                        i -> [w5730]
                        n1107 = case shown="0, Default" w5730 {
                          tunnel: [w5735 w5739] -> w5729
                          frame 0, Default {
                            n1108 = Select(t=1, s="Freq 3", f=0) -> (s? t:f=w5735:i32)
                          }
                          frame 1 {
                            n1109 = Select(t=2, s="Duty", f=0) -> (s? t:f=w5739:i32)
                          }
                        }
                        n1110 = case shown="2" w5729 {
                          tunnel: w5728 -> [w5745 w5752 w5763]
                          tunnel: w5727 -> [w5744 w5751 w5766]
                          tunnel: w5726 -> [w5743 w5750 w5768]
                          tunnel: [w5745 w5749 w5762] -> w5734
                          tunnel: [w5744 w5748 w5765] -> w5733
                          tunnel: [w5743 w5747 w5767] -> w5732
                          tunnel: w5731 -> [_ w5746 w5764]
                          frame 0, Default {
                          }
                          frame 1 {
                            n1111 = case shown="\"ULx\", Default" w5746 {
                              tunnel: w5751 -> [w5755 w5761]
                              tunnel: [w5756 w5759] -> w5747
                              tunnel: [w5754 w5761] -> w5748
                              tunnel: [w5758 w5760] -> w5749
                              tunnel: w5752 -> [w5758 w5760]
                              tunnel: w5750 -> [w5757 w5759]
                              frame "ULx", Default {
                                n1112 = property class="IOTask"(reference=w5755, error in=w5757, "Channel.CO.Pulse.Frequency.Frequency"="Frequency") -> (reference out=w5754:refnum<k24>, error out=w5756:errorcluster)
                              }
                              frame "DAQmx" {
                              }
                            }
                          }
                          frame 2 {
                            n1113 = case shown="\"ULx\", Default" w5764 {
                              tunnel: w5768 -> [w5772 w5776]
                              tunnel: [w5771 w5776] -> w5767
                              tunnel: w5766 -> [w5770 w5777]
                              tunnel: [w5769 w5777] -> w5765
                              tunnel: w5763 -> [w5774 w5775]
                              tunnel: [w5774 w5775] -> w5762
                              frame "ULx", Default {
                                n1114 = property class="IOTask"(reference=w5770, error in=w5772, "Channel.CO.Pulse.Frequency.DutyCycle"="DutyCycle") -> (reference out=w5769:refnum<k24>, error out=w5771:errorcluster)
                              }
                              frame "DAQmx" {
                              }
                            }
                          }
                        }
                      }
                    }
                  }
                }
              }
            }
          }
          n1115 = local write "Props"(w3935) -> ()
        }
        frame 14 {
          # "Task Control"
          n1116 = for {
            N: 5 -> [_]
            tunnel: w5779 -> [w5790]
            tunnel: [FALSE] -> w5780
            n1117 = Wait Until Next ms Multiple(millisecond multiple=w5790) -> ()  [unwired: 1 out]
            "TC" <- TRUE
          }
          n1118 = local write "TC"(w5780) -> ()
          n1119 = case shown="\"ULx\", Default" w5784 {
            tunnel: w5786 -> [w5793 w5800]
            tunnel: w5785 -> [w5792 w5799]
            tunnel: [w5792 w5798] -> w5782
            tunnel: w5788 -> [w5794 w5797]
            tunnel: [w5794 w5795] -> w5787
            tunnel: [w5793 w5800] -> w5783
            frame "ULx", Default {
            }
            frame "DAQmx" {
              n1120 = call <vilib>:"DAQmx Control Task.vi"("task/channels in"=w5797, "action"="Task Control Action", "error in"=w5799) -> ("task out"=w5795:refnum<k21>, "error out"=w5798:errorcluster)  [unwired: 11 in]
            }
          }
          n1121 = local write "NI\nTC"(FALSE ("TC")) -> ()
        }
      }
      n1122 = Select(t=u32 20 ("millisecond multiple"), s=w25, f="Loop") -> (s? t:f=w27:u32)
      n1123 = Wait Until Next ms Multiple(millisecond multiple=w27) -> ()  [unwired: 1 out]
    }
  }
  n1124 = local write "message 2"("") -> ()
  n1125 = local write "Task"(0 ("Task")) -> ()
  n1126 = local write "Task Cleared"(w5) -> ()
  n1127 = local write "Task Stopped"(w5) -> ()
  n1128 = call <vilib>:"DAQmx Clear Task.vi"("task in"=w3) -> ()  [unwired: 14 in, 1 out]
  n1129 = call <vilib>:"ULx Clear Task.vi"("task in"=w2) -> ()  [unwired: 14 in, 1 out]
  n1130 = local write "stop"(w6) -> ()
